vi "PDE_Cal Start Idx and Length.vi"(9 "# of points":i32, 10 "end type":T1 items=["Dirichlet", "Neumann"], 11 "start type":T1 items=["Dirichlet", "Neumann"]) -> (2 "length":i32, 3 "start index":i32)   [LabVIEW 2020, in "NI_PDE.lvlib"]
uses:
  <vilib>/gmath/NI_PDE.lvlib
  <vilib>/gmath/pde.llb/Common/PDE_BC Type.ctl
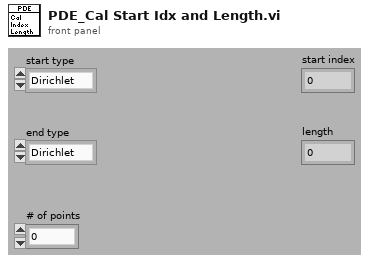
[diagram p1: front panel]
types:
  T1 = typedef "NI_PDE.lvlib/PDE_BC Type.ctl" = i32
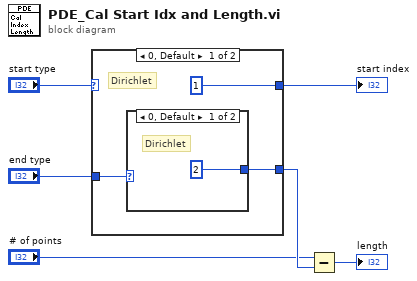
[diagram p0: block diagram]
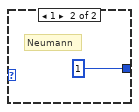
[diagram p2: hidden frame]
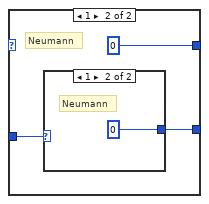
[diagram p3: hidden frame]
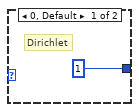
[diagram p4: hidden frame]
diagram:
  n1 = case shown="0, Default" "start type" {
    tunnel: [1 0] -> w6
    tunnel: "end type" -> [w8 w13]
    tunnel: [w7 w12] -> w5
    frame 0, Default {
      # "Dirichlet"
      n2 = case shown="0, Default" w8 {
        tunnel: [2 1] -> w7
        frame 0, Default {
          # "Dirichlet"
        }
        frame 1 {
          # "Neumann"
        }
      }
    }
    frame 1 {
      # "Neumann"
      n3 = case shown="1" w13 {
        tunnel: [1 0] -> w12
        frame 0, Default {
          # "Dirichlet"
        }
        frame 1 {
          # "Neumann"
        }
      }
    }
  }
  "start index" <- w6
  n4 = Subtract(x="# of points", y=w5) -> (x-y=→"length":i32)
